vi "数组的基本使用2.vi"() -> ()   [LabVIEW 2018]
panel:
  in  "维度 列":dbl
  in  "维度 行":dbl
  out "输出数组 2":dbl[][](array[numeric])
  in  "原数组 11":dbl[][](array[numeric])
  out "数组元素之积":dbl
  out "数组元素之和":dbl
  in  "原数组 10":dbl[](array[numeric])
  out "原数组 9":dbl[][](array[numeric])
  out "转置数组":dbl[][](array[numeric])
  in  "搜索起始位置索引":dbl
  out "位置":dbl
  in  "元素":dbl
  out "原数组 8":dbl[](array[numeric])
  out "原数组 7":dbl[](array[numeric])
  out "新数组 4":dbl[](array[numeric])
  in  "索引 2":dbl
  out "新数组 3":dbl[](array[numeric])
  out "新数组 2":dbl[](array[numeric])
  out "原数组 6":dbl[](array[numeric])
  in  "索引":dbl
  out "新数组":dbl[](array[numeric])
  in  "要插入的数组":dbl[](array[numeric])
  out "原数组 5":dbl[](array[numeric])
  in  "长度-行数量":dbl
  in  "索引-行索引":dbl
  out "数组 3":dbl[][](array[numeric])
  out "原数组 4":dbl[][](array[numeric])
  in  "输入数值":dbl
  out "输出数组":dbl[][](array[numeric])
  in  "列索引 2":dbl
  in  "行索引 2":dbl
  out "数值 2":dbl
  in  "列索引":dbl
  in  "行索引":dbl
  out "原数组 3":dbl[][](array[numeric])
  in  "长度-行数量":dbl
  in  "索引-行索引：表示第几行":dbl
  out "原数组 2":dbl[][](array[numeric])
  out "被删除后的数组":dbl[][](array[numeric])
  out "被删除的数组":dbl[][](array[numeric])
  out "最小值位置索引":dbl[](array[numeric])
  out "最大值位置索引":dbl[](array[numeric])
  out "最小值":dbl
  out "最大值":dbl
  out "一维数组成员数":dbl
  out "二维数组成员个数":dbl[](array[numeric])
  out "数组 2":dbl[][](array[numeric])
  out "字符串 2":string[](array[string])
  out "数值":dbl[](array[numeric])
  out "数组":string[][](array[string])
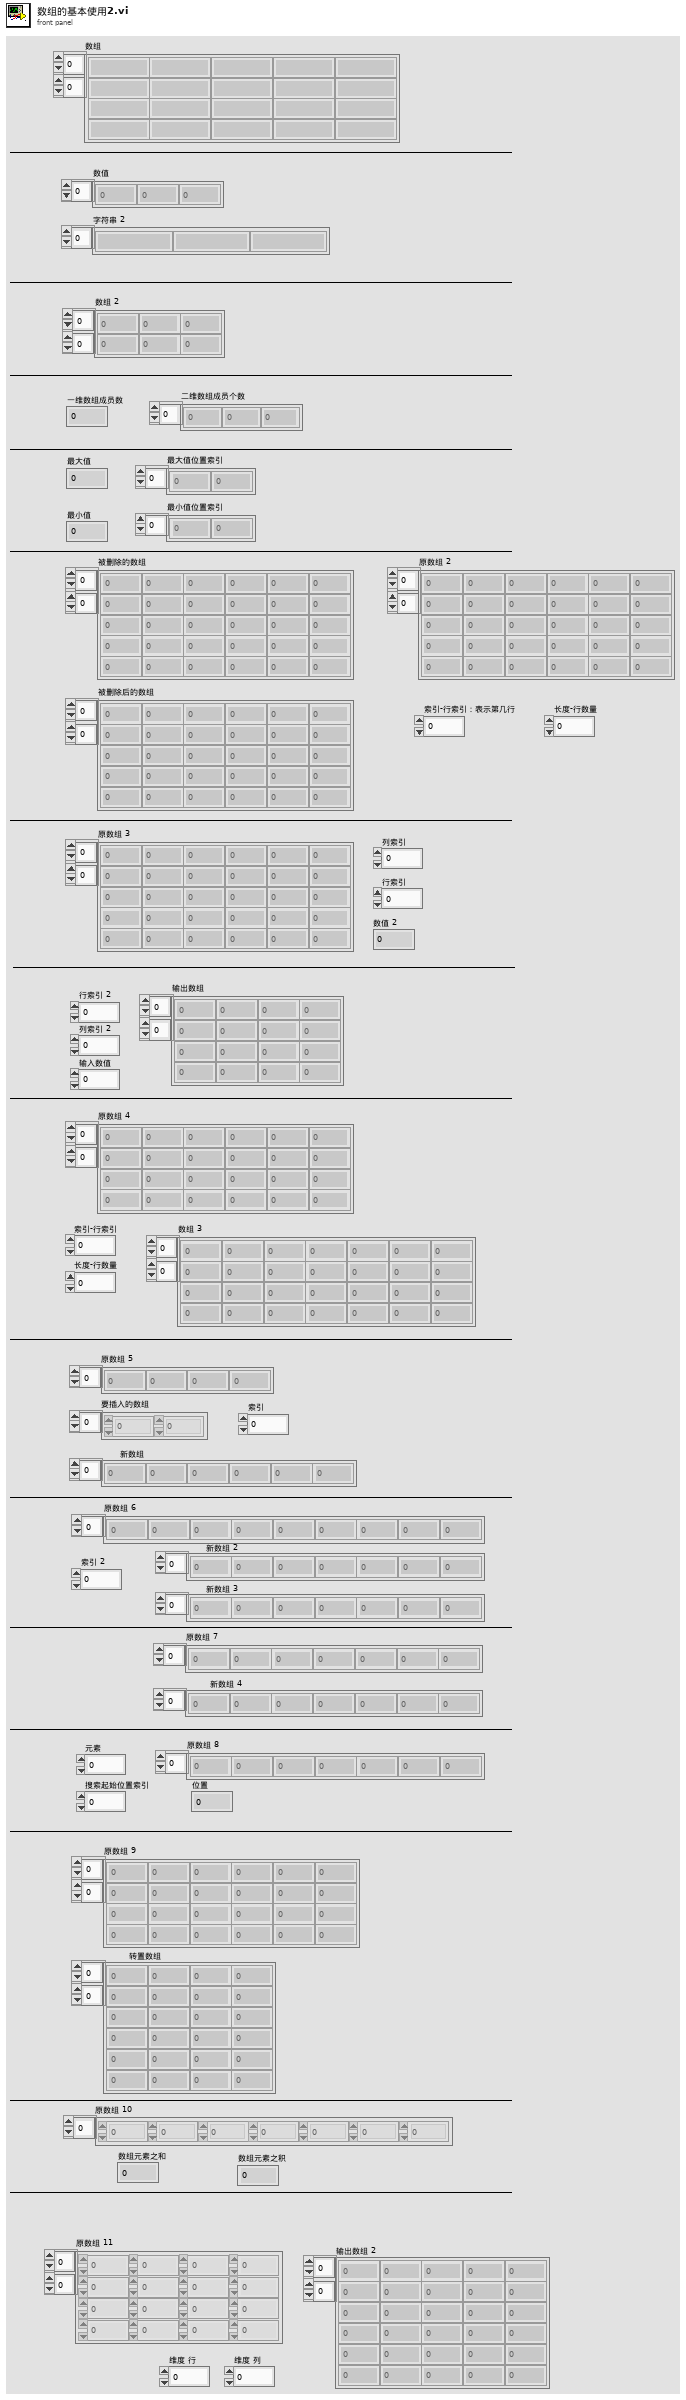
[diagram p1: front panel]
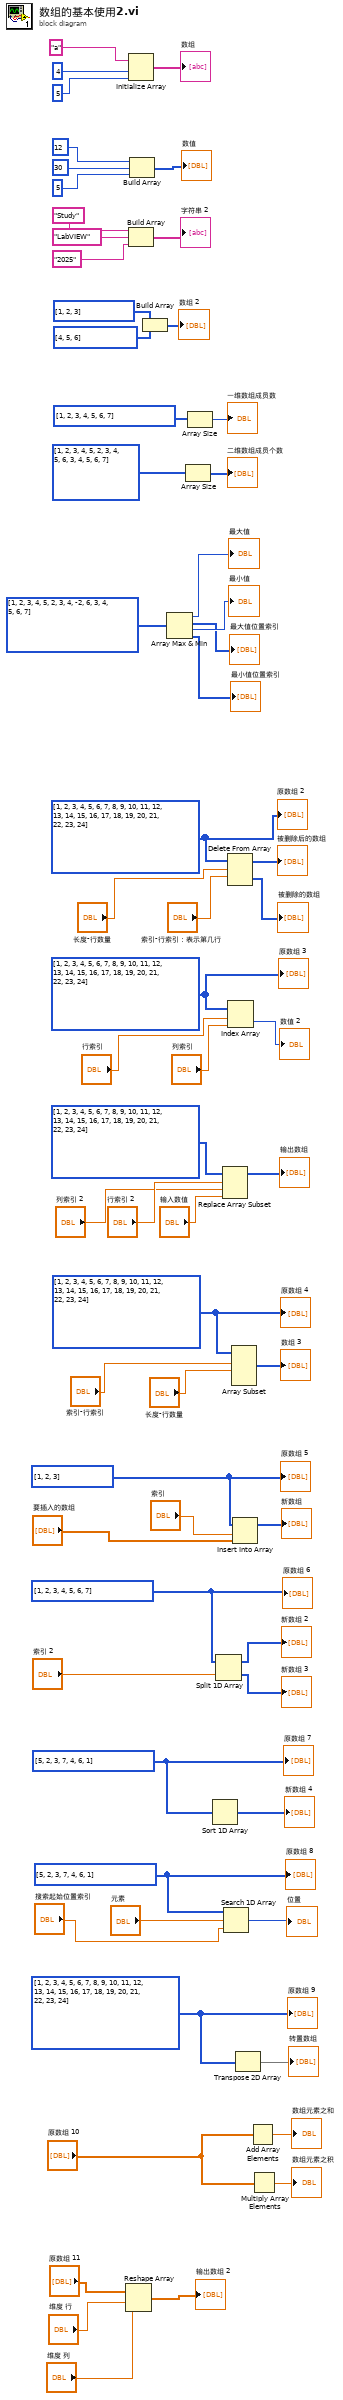
[diagram p0: block diagram]
diagram:
  w8 = i32[][] [[1, 2, 3, 4, 5, 6], [7, 8, 9, 10, 11, 12], [13, 14, 15, 16, 17, 18], [19, 20, 21, 22, 23, 24]]
  w12 = i32[] [5, 2, 3, 7, 4, 6, 1]
  w14 = i32[] [5, 2, 3, 7, 4, 6, 1]
  w16 = i32[] [1, 2, 3, 4, 5, 6, 7]
  w20 = i32[] [1, 2, 3]
  w27 = i32[][] [[1, 2, 3, 4, 5, 6], [7, 8, 9, 10, 11, 12], [13, 14, 15, 16, 17, 18], [19, 20, 21, 22, 23, 24]]
  w36 = i32[][] [[1, 2, 3, 4, 5, 6], [7, 8, 9, 10, 11, 12], [13, 14, 15, 16, 17, 18], [19, 20, 21, 22, 23, 24]]
  w40 = i32[][] [[1, 2, 3, 4, 5, 6], [7, 8, 9, 10, 11, 12], [13, 14, 15, 16, 17, 18], [19, 20, 21, 22, 23, 24]]
  n1 = Reshape Array("原数组 11", "维度 行", "维度 列") -> (→"输出数组 2":dbl[][])
  n2 = Initialize Array("a", 4, 5) -> (→"数组":string[][])
  n3 = Build Array("Study", "LabVIEW", "2025") -> (→"字符串 2":string[])
  n4 = Build Array(12, 30, 5) -> (→"数值":i32[])
  n5 = Build Array(i32[] [1, 2, 3], i32[] [4, 5, 6]) -> (→"数组 2":i32[][])
  n6 = Array Max & Min(array=i32[][] [[1, 2, 3, 4, 5], [2, 3, 4, -2, 6], [3, 4, 5, 6, 7]]) -> (max value=→"最大值":i32, max index (indices)=→"最大值位置索引":i32[], min value=→"最小值":i32, min index (indices)=→"最小值位置索引":i32[])
  n7 = Array Size(array=i32[][] [[1, 2, 3, 4, 5], [2, 3, 4, 5, 6], [3, 4, 5, 6, 7]]) -> (size(s)=→"二维数组成员个数":i32[])
  n8 = Array Size(array=i32[] [1, 2, 3, 4, 5, 6, 7]) -> (size(s)=→"一维数组成员数":i32)
  n9 = Sort 1D Array(array=w14) -> (sorted array=→"新数组 4":i32[])
  n10 = Split 1D Array(array=w16, index="索引 2") -> (first subarray=→"新数组 2":i32[], second subarray=→"新数组 3":i32[])
  n11 = Replace Array Subset(array=i32[][] [[1, 2, 3, 4, 5, 6], [7, 8, 9, 10, 11, 12], [13, 14, 15, 16, 17, 18], [19, 20, 21, 22, 23, 24]], new element="输入数值", index (row)="行索引 2", index (col)="列索引 2") -> (→"输出数组":i32[][])
  n12 = Search 1D Array(1D array=w12, element="元素", start index (0)="搜索起始位置索引") -> (index of element=→"位置":i32)
  n13 = Delete From Array(array=w40, length="长度-行数量", index (row)="索引-行索引：表示第几行") -> (deleted portion=→"被删除的数组":i32[][], array with subset deleted=→"被删除后的数组":i32[][])  [unwired: 1 in]
  n14 = Index Array(array=w36, index (row)="行索引", index (col)="列索引") -> (element=→"数值 2":i32)
  n15 = Array Subset(array=w27, index (row)="索引-行索引", length (row)="长度-行数量") -> (→"数组 3":i32[][])  [unwired: 2 in]
  n16 = Insert Into Array(array=w20, index="索引", new element="要插入的数组") -> (→"新数组":i32[])
  n17 = Transpose 2D Array(2D array=w8) -> (transposed array=→"转置数组":i32[][])
  n18 = Add Array Elements(numeric array="原数组 10") -> (sum=→"数组元素之和":dbl)
  n19 = Multiply Array Elements(1:"原数组 10") -> (0:→"数组元素之积":dbl)
  "原数组 2" <- w40
  "原数组 3" <- w36
  "原数组 4" <- w27
  "原数组 5" <- w20
  "原数组 6" <- w16
  "原数组 7" <- w14
  "原数组 8" <- w12
  "原数组 9" <- w8
